vi "DataLog Set Tag Value_srv.vi"(0 "tag":string, 7 "value":dbl, 11 "certificate":string) -> (15 "error out":errorcluster)   [LabVIEW 2012]
uses:
  clientsrv/typedefs/t_ClientSrv Access Levels.ctl
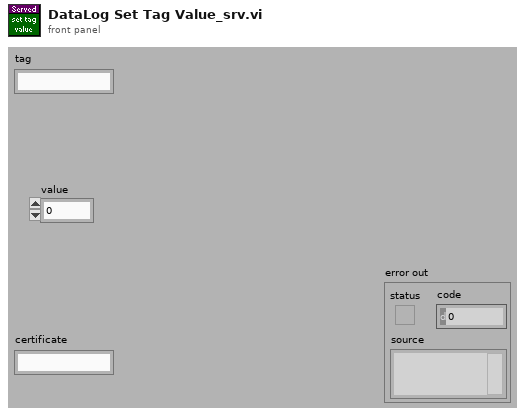
[diagram p1: front panel]
types:
  T1 = typedef "t_ClientSrv Access Levels.ctl" = enum16{"observer", "operator", "local"}
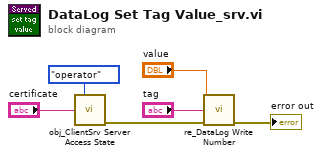
[diagram p0: block diagram]
diagram:
  n1 = call "obj_ClientSrv Server Access State.vi"("access level"=t_ClientSrv_Access_Levels."operator", "certificate in"="certificate") -> ("error out"=w4:errorcluster)  [unwired: 11 in, 2 out]
  n2 = call "re_DataLog Write Number.vi"("number"="value", "tag"="tag", "error in (no error)"=w4) -> ("error out"=→"error out":errorcluster)  [unwired: 11 in, 1 out]
